vi "Get Color.vi"(8 "error in (no error)":errorcluster, 11 "ColorSensorDevRef":T1={"I2CDevRef"={"DevStatus"={"status"=FALSE, "code"=0, "source"=""}, "Device Address"=0, "Handle"=0, "I2C Bus"=enum."Invalid"}, "Confidence Threshold"=0.95} {"I2CDevRef"."Device Address" format="%.0x"}) -> (0 "error out":errorcluster, 1 "Confidence":dbl, 2 "Color":T4, 3 "ColorSensorDevRef out":T1={"I2CDevRef"={"DevStatus"={"status"=FALSE, "code"=0, "source"=""}, "Device Address"=0, "Handle"=0, "I2C Bus"=enum."Invalid"}, "Confidence Threshold"=0.95} {"I2CDevRef"."Device Address" format="%.0x"})   [LabVIEW 2018, in "ColorSensor.lvlib"]
uses:
  ColorSensor.lvlib
  TypeDef/ColorSensorDevRef.ctl
  <vilib>/Rock Robotics/WPI/I2C/WPI_I2CDevRef.ctl
  <vilib>/Rock Robotics/SystemInterfaces/i2clib/i2c_bus.ctl
  TypeDef/Color.ctl
  TypeDef/CalibCoeff.ctl
  TypeDef/NormColorValues.ctl
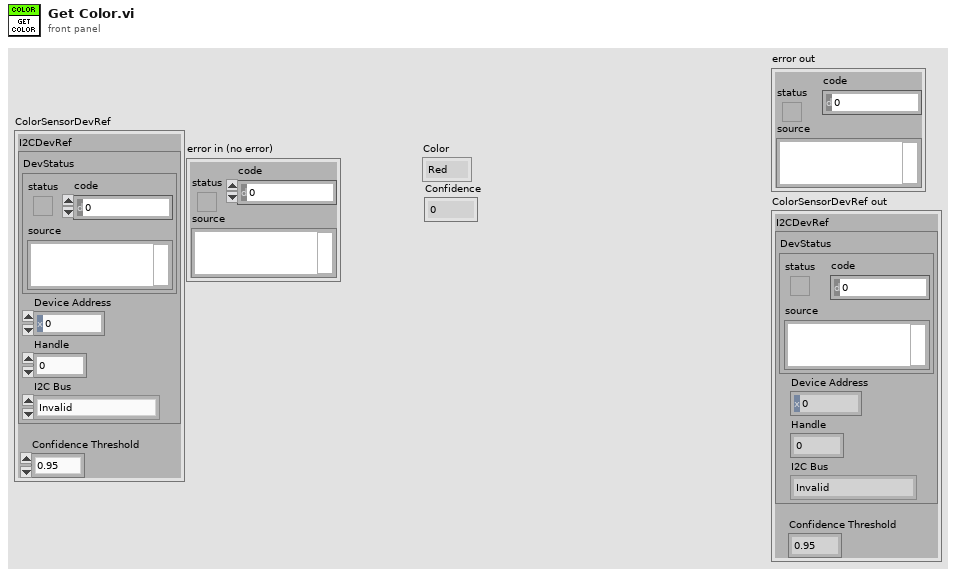
[diagram p1: front panel]
types:
  T1 = typedef "ColorSensor.lvlib/ColorSensorDevRef.ctl" = cluster{"I2CDevRef":T2, "Confidence Threshold":dbl}
  T2 = typedef "WPI_I2CDevRef.ctl" = cluster{"DevStatus":errorcluster, "Device Address":u8, "Handle":i32, "I2C Bus":T3}
  T3 = typedef "i2c_bus.ctl" = enum16{"I2C On-Board", "I2C MXP", "Invalid"}
  T4 = typedef "ColorSensor.lvlib/Color.ctl" = enum16{"Red", "Green", "Blue", "Yellow", "Unknown"}
  T5 = typedef "ColorSensor.lvlib/CalibCoeff.ctl" = cluster{"NormColorValues":T6, "Color":T4}
  T6 = typedef "ColorSensor.lvlib/NormColorValues.ctl" = cluster{"Blue":dbl, "Green":dbl, "Red":dbl, "IR":dbl}
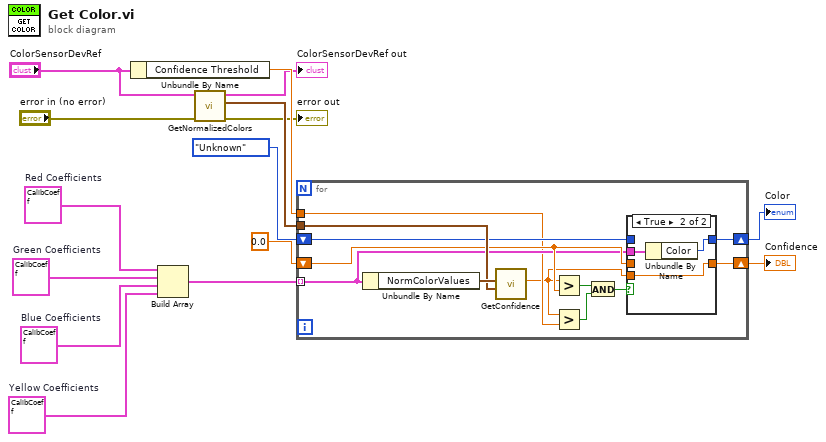
[diagram p0: block diagram]
diagram:
  w11 = T5 {"NormColorValues"={"Blue"=0.112, "Green"=0.529, "Red"=0.349, "IR"=0.01}, "Color"=enum."Yellow"}  # Yellow Coefficients
  w12 = T5 {"NormColorValues"={"Blue"=0.435, "Green"=0.415, "Red"=0.133, "IR"=0.017}, "Color"=enum."Blue"}  # Blue Coefficients
  w13 = T5 {"NormColorValues"={"Blue"=0.241, "Green"=0.548, "Red"=0.189, "IR"=0.022}, "Color"=enum."Green"}  # Green Coefficients
  w14 = T5 {"NormColorValues"={"Blue"=0.117, "Green"=0.319, "Red"=0.54, "IR"=0.024}, "Color"=enum."Red"}  # Red Coefficients
  n1 = Unbundle By Name("ColorSensorDevRef") -> ("Confidence Threshold"=w3:dbl)
  n2 = Build Array(w14, w13, w12, w11) -> (w10:T5[])
  n3 = call "GetNormalizedColors.vi"("error in (no error)"="error in (no error)", "ColorSensorDevRef"="ColorSensorDevRef") -> ("error out"=→"error out":errorcluster, "Normalized Colors"=w9:T6, "ColorSensorDevRef out"=→"ColorSensorDevRef out":T1)  [unwired: 7 in]
  n4 = for {
    tunnel: w10 -> [w23] mode=indexing
    tunnel: w9 -> [w26]
    shift-right: [w24] -> w5
    shift-left: 0.0 ("y") -> [w25]
    shift-right: [w22] -> w6
    shift-left: Color."Unknown" ("Color") -> [w21]
    tunnel: w3 -> [w19]
    n5 = Unbundle By Name(w23) -> ("NormColorValues"=w27:T6)
    n6 = call "GetConfidence.vi"("Measured Values"=w26, "Calib Coefficients"=w27) -> ("Confidence"=w18:dbl)  [unwired: 9 in]
    n7 = Greater?(x=w18, y=w25) -> (0:w20:bool)
    n8 = Greater?(x=w18, y=w19) -> (0:w17:bool)
    n9 = And(x=w20, y=w17) -> (x .and. y?=w16:bool)
    n10 = case shown="True" w16 {
      tunnel: w18 -> [_ w32]
      tunnel: w25 -> [w29 _]
      tunnel: [w29 w32] -> w24
      tunnel: w23 -> [_ w31]
      tunnel: [w28 w30] -> w22
      tunnel: w21 -> [w28 _]
      frame False {
      }
      frame True {
        n11 = Unbundle By Name(w31) -> ("Color"=w30:T4)
      }
    }
  }
  "Color" <- w6
  "Confidence" <- w5
